vi "Labview TimeStamp to BD Timestamp.vi"(1 "Data/hora":timestamp) -> (0 "date/time string":string)   [LabVIEW 2020, in "PostgreSQL Driver.lvlib"]
uses:
  Type Defs/Time Format String.ctl
  PostgreSQL Driver.lvlib
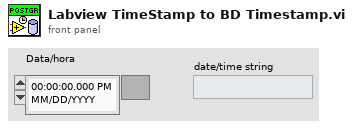
[diagram p1: front panel]
types:
  T1 = typedef "PostgreSQL Driver.lvlib/Time Format String.ctl" = string
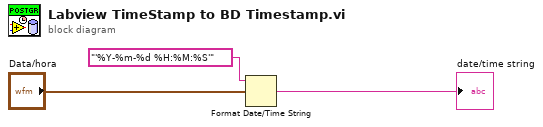
[diagram p0: block diagram]
diagram:
  n1 = Format Date/Time String(time format string (%c)=T1 "'%Y-%m-%d %H:%M:%S'", seconds (now)="Data/hora") -> (date/time string=→"date/time string":string)  [unwired: 1 in]
